vi "Get Clock (Calendar).vi"(0 "VISA resource name":refnum<visa-resource-name>, 11 "error in (no error)":errorcluster) -> (3 "Hour":i32, 4 "VISA resource name out":refnum<visa-resource-name>, 6 "Minute":i32, 8 "Second":i32, 10 "Day":i32, 13 "Year":i32, 14 "Month":i32, 15 "error out":errorcluster)   [LabVIEW 2011, in "Fluke 5XXX Series Multicalibrators.lvlib"]
doc: "This VI returns the instrument's internal clock and calendar settings.\n\nNote:\n\nThis VI is available only for instrument models 5520A, 5700A, 5720A and 57LFC."
uses:
  Fluke 5XXX Series Multicalibrators.lvlib
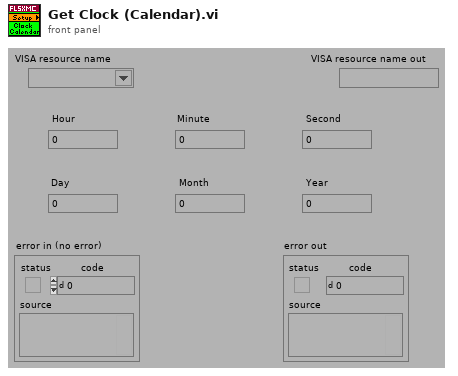
[diagram p1: front panel]
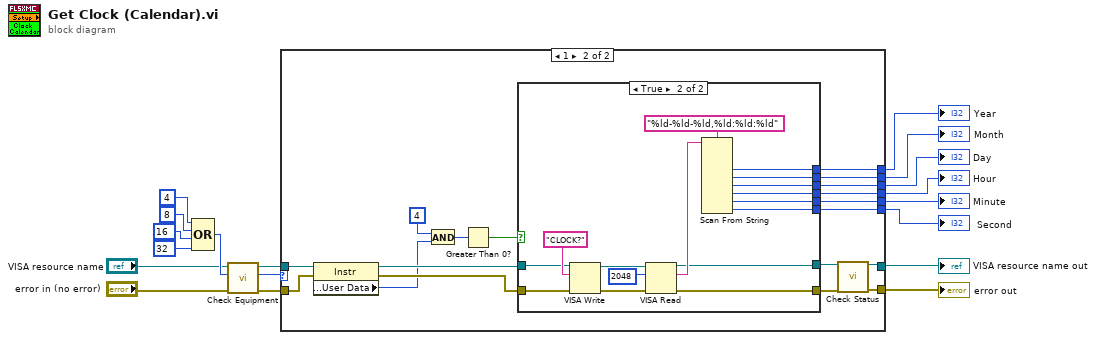
[diagram p0: block diagram]
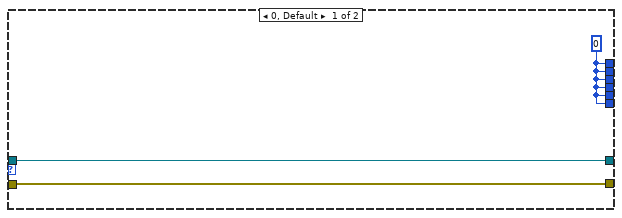
[diagram p2: hidden frame]
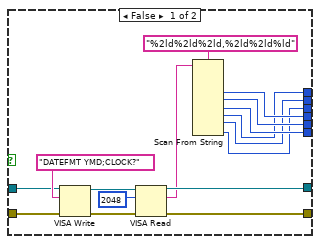
[diagram p3: hidden frame]
diagram:
  n1 = Compound Arithmetic op=OR(4 ("Numeric"), 8 ("Numeric"), 16 ("Numeric"), 32 ("Numeric")) -> (w12:i32)
  n2 = call "Check Equipment.vi"("error in (no error)"="error in (no error)", "Bit Mask"=w12, "VISA resource name"="VISA resource name") -> ("error out"=w15:errorcluster, "Present?"=w13:u32, "VISA resource name out"=w14:refnum<visa-resource-name>)  [unwired: 6 in]
  n3 = case shown="1" w13 {
    tunnel: [w20 w38] -> w11
    tunnel: w15 -> [w21 w28]
    tunnel: w14 -> [w20 w29]
    tunnel: [w21 w39] -> w10
    tunnel: [w19 w35] -> w7
    tunnel: [w19 w34] -> w6
    tunnel: [w19 w33] -> w5
    tunnel: [w19 w32] -> w4
    tunnel: [w19 w31] -> w3
    tunnel: [w19 w30] -> w2
    frame 0, Default {
      w19 = 0
    }
    frame 1 {
      n4 = property class="Instr"(reference=w29, error in=w28) -> (reference out=w27:refnum<visa-resource-name>, error out=w26:errorcluster, "General Settings:User Data"=w25:u32)
      n5 = And(x=u32 4 ("Numeric"), y=w25) -> (x .and. y?=w23:u32)
      n6 = Greater Than 0?(x=w23) -> (x > 0?=w22:bool)
      n7 = case shown="True" w22 {
        tunnel: w26 -> [w47 w65]
        tunnel: [w50 w64] -> w37
        tunnel: [w49 w63] -> w36
        tunnel: w27 -> [w48 w62]
        tunnel: [w43 w61] -> w35
        tunnel: [w42 w60] -> w34
        tunnel: [w41 w59] -> w33
        tunnel: [w46 w58] -> w32
        tunnel: [w45 w57] -> w31
        tunnel: [w44 w56] -> w30
        frame False {
          n8 = VISA Write(VISA resource name=w48, write buffer="DATEFMT YMD;CLOCK?", error in (no error)=w47) -> (VISA resource name out=w53:refnum<visa-resource-name>, error out=w52:errorcluster)  [unwired: 1 out]
          n9 = VISA Read(VISA resource name=w53, byte count=u32 2048 ("byte count (0)"), error in (no error)=w52) -> (VISA resource name out=w49:refnum<visa-resource-name>, read buffer=w40:string, error out=w50:errorcluster)  [unwired: 1 out]
          n10 = Scan From String(format string="%2ld%2ld%2ld,%2ld%2ld%ld", input string=w40) -> (output 1=w46:i32, output 2=w45:i32, output 3=w44:i32, output 4=w43:i32, output 5=w42:i32, output 6=w41:i32)  [unwired: 8 in, 3 out]
        }
        frame True {
          n11 = VISA Write(VISA resource name=w62, write buffer="CLOCK?", error in (no error)=w65) -> (VISA resource name out=w69:refnum<visa-resource-name>, error out=w68:errorcluster)  [unwired: 1 out]
          n12 = VISA Read(VISA resource name=w69, byte count=u32 2048 ("byte count (0)"), error in (no error)=w68) -> (VISA resource name out=w63:refnum<visa-resource-name>, read buffer=w66:string, error out=w64:errorcluster)  [unwired: 1 out]
          n13 = Scan From String(format string="%ld-%ld-%ld,%ld:%ld:%ld", input string=w66) -> (output 1=w61:i32, output 2=w60:i32, output 3=w59:i32, output 4=w58:i32, output 5=w57:i32, output 6=w56:i32)  [unwired: 8 in, 3 out]
        }
      }
      n14 = call "Check Status.vi"("VISA resource name"=w36, "error in (no error)"=w37) -> ("VISA resource name out"=w38:refnum<visa-resource-name>, "error out"=w39:errorcluster)  [unwired: 12 in]
    }
  }
  "Hour" <- w4
  "Minute" <- w3
  "Second" <- w2
  "Day" <- w5
  "Month" <- w6
  "Year" <- w7
  "VISA resource name out" <- w11
  "error out" <- w10
